vi "Paint Demo.vi"() -> ()   [LabVIEW 2011]
doc: "This VI shows how to implement an XControl. The Paint XControl included with this example demonstrates how to use some of the picture functions available in a LabVIEW XControl. The XControl allows you to paint objects such as lines, circles, and text into a picture control. The Paint XControl then outputs the painted image."
uses:
  xcontrol vis/paint Xcontrol.xctl
panel:
  in  "Tab Control":enum32{"Paint XControl", "Mirror Image"}(tab)
  in  "Paint XControl":picture(xcontrol)
  out "Mirror Image":picture
  in  "stop":bool
  # "Directions:\n1. Run the VI. \n2. Select a drawing tool and set the line style and color you want to use. Place a checkmark in the Fill Shapes checkbox to color-fill the circle and square shapes when you draw them.\n3. Right-click the canvas to open a shortcut menu from which you can undo the last action, save the image, import a new image, or clear the canvas.\n4. Select the Mirror Image tab to verify the output of the Paint XControl.\n\nNote: You also can use the XControl as an indicator if you wish to draw on top of an existing image."
  # "Select Help»Show Context Help and move the cursor over the VI icon to display help for this VI."
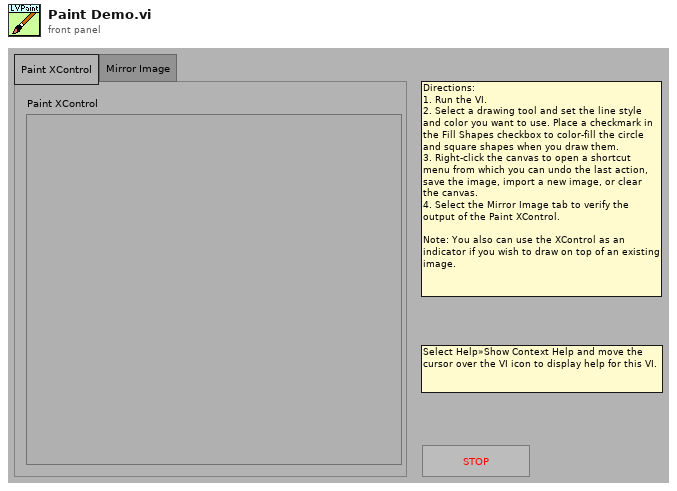
[diagram p1: front panel]
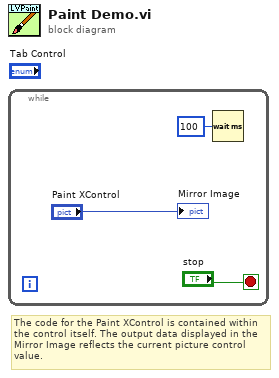
[diagram p0: block diagram]
diagram:
  # "The code for the Paint XControl is contained within\nthe control itself. The output data displayed in the Mirror Image reflects the current picture control value."
  n1 = while {
    stop <- "stop" stop-if-true
    n2 = Wait (ms)(milliseconds to wait=u32 100) -> ()  [unwired: 1 out]
    "Mirror Image" <- "Paint XControl"
  }
